vi "TDTSyn-Init ActiveX.vi"(0 "Init TTankX?":bool=TRUE, 5 "Init TDevAccX?":bool=TRUE, 11 "error in (no error)":errorcluster) -> (4 "TTANKXLib.TTankX":refnum<k7>, 6 "TDEVACCXLib.TDevAccX":refnum<k7>, 15 "error out":errorcluster)   [LabVIEW 2020]
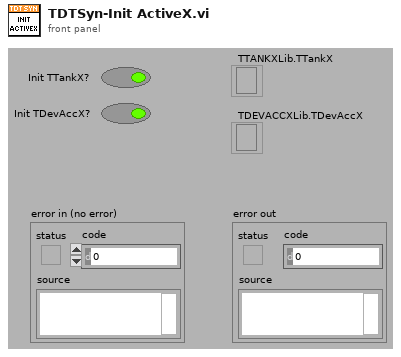
[diagram p1: front panel]
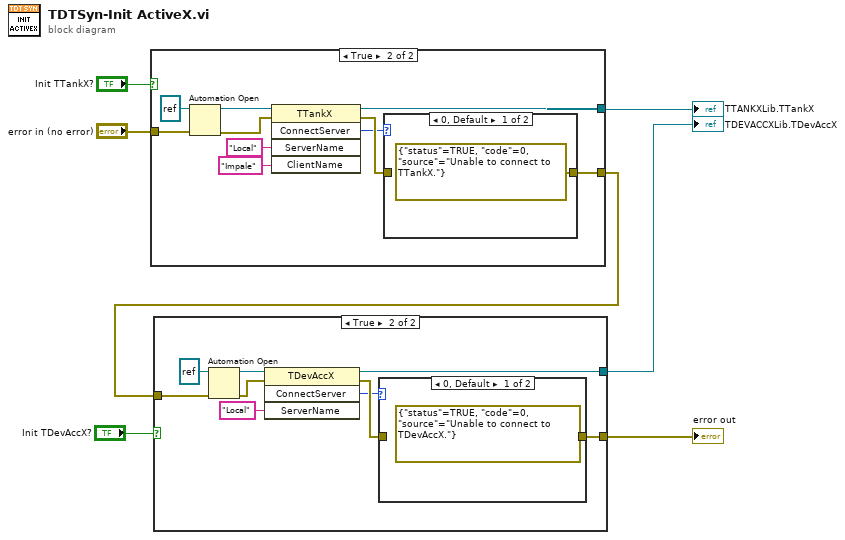
[diagram p0: block diagram]
diagram:
  n1 = case shown="True" "Init TTankX?" {
    tunnel: [w8 w18] -> w6
    tunnel: [_ w15] -> w4
    tunnel: "error in (no error)" -> [w8 w9]
    frame False {
    }
    frame True {
      n2 = Automation Open(error in (no error)=w9, Automation Refnum=refnum<k7> refnum ("TTANKXLib.TTankX")) -> (Automation Refnum=w11:refnum<k7>, error out=w12:errorcluster)  [unwired: 2 in]
      n3 = invoke class="TTankX" method="ConnectServer"(reference=w11, error in=w12, "ServerName"="Local", "ClientName"="Impale") -> (reference out=w15:refnum<k7>, error out=w17:errorcluster, "ConnectServer"=w16:i32)  [unwired: 1 in, 2 out]
      n4 = case shown="0, Default" w16 {
        tunnel: w17 -> [_ w20]
        tunnel: [errorcluster {"status"=TRUE, "code"=0, "source"="Unable to connect to TTankX."} ("error out") w20] -> w18
        frame 0, Default {
        }
        frame 1 {
        }
      }
    }
  }
  "TTANKXLib.TTankX" <- w4
  n5 = case shown="True" "Init TDevAccX?" {
    tunnel: [w21 w25] -> w7
    tunnel: w6 -> [w21 w23]
    tunnel: [_ w22] -> w5
    frame False {
    }
    frame True {
      n6 = Automation Open(error in (no error)=w23, Automation Refnum=refnum<k7> refnum ("TDEVACCXLib.TDevAccX")) -> (Automation Refnum=w28:refnum<k7>, error out=w29:errorcluster)  [unwired: 2 in]
      n7 = invoke class="TDevAccX" method="ConnectServer"(reference=w28, error in=w29, "ServerName"="Local") -> (reference out=w22:refnum<k7>, error out=w26:errorcluster, "ConnectServer"=w24:i32)  [unwired: 1 in, 1 out]
      n8 = case shown="0, Default" w24 {
        tunnel: w26 -> [_ w32]
        tunnel: [errorcluster {"status"=TRUE, "code"=0, "source"="Unable to connect to TDevAccX."} ("error out") w32] -> w25
        frame 0, Default {
        }
        frame 1 {
        }
      }
    }
  }
  "error out" <- w7
  "TDEVACCXLib.TDevAccX" <- w5
